vi "Configure DC Power Voltage.vi"(0 "VISA resource name":refnum<visa-resource-name>, 1 "DC Power Voltage (0 V)":dbl format="%^#_9g", 5 "Enable DC Power Output (Disable)":bool, 7 "Max Power Voltage Limit (16 V)":dbl=16.0 format="%^#_9g", 9 "Min Power Voltage Limit (0 V)":dbl format="%^#_9g", 11 "error in (no error)":errorcluster, 12 "DC Power Delay (100E-3 s)":dbl=0.1 format="%^#_9g") -> (4 "VISA resource name out":refnum<visa-resource-name>, 15 "error out":errorcluster)   [LabVIEW 2011, in "Agilent E5052X.lvlib"]
doc: "Configures the instrument's DC Power settings and how it will be applied to the DUT interface. \n\n<b>Note: </b>\n\nThis VI can be used for voltage control oscillator measurements."
uses:
  Agilent E5052X.lvlib
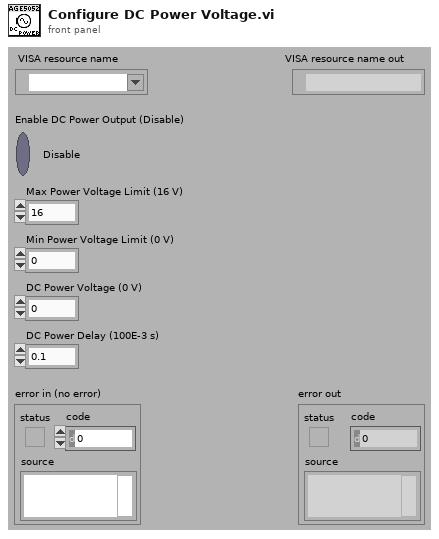
[diagram p1: front panel]
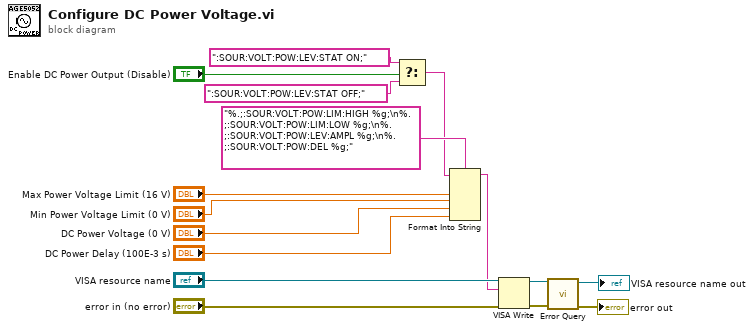
[diagram p0: block diagram]
diagram:
  n1 = Select(t=":SOUR:VOLT:POW:LEV:STAT ON;", s="Enable DC Power Output (Disable)", f=":SOUR:VOLT:POW:LEV:STAT OFF;") -> (s? t:f=w2:string)
  n2 = Format Into String(format string="%.;:SOUR:VOLT:POW:LIM:HIGH %g;\n%.;:SOUR:VOLT:POW:LIM:LOW %g;\n%.;:SOUR:VOLT:POW:LEV:AMPL %g;\n%.;:SOUR:VOLT:POW:DEL %g;", initial string=w2, "Max Power Voltage Limit (16 V)", "Min Power Voltage Limit (0 V)", "DC Power Voltage (0 V)", "DC Power Delay (100E-3 s)") -> (resulting string=w1:string)  [unwired: 1 in, 1 out]
  n3 = VISA Write(VISA resource name="VISA resource name", write buffer=w1, error in (no error)="error in (no error)") -> (VISA resource name out=w9:refnum<visa-resource-name>, error out=w8:errorcluster)  [unwired: 1 out]
  n4 = call "Error Query.vi"("error in (no error)"=w8, "VISA resource name"=w9) -> ("error out"=→"error out":errorcluster, "VISA resource name out"=→"VISA resource name out":refnum<visa-resource-name>)  [unwired: 6 in, 2 out]
